vi "Inverse Filter Demo-1.vi"() -> ()   [LabVIEW 2015]
uses:
  Utility VIs/Math VIs/FFT x(t) to dB,Degrees (1D).vi
  Utility VIs/Math VIs/Linear to dB (array).vi
  <vilib>/Analysis/NI_AALBase.lvlib
  Utility VIs/Math VIs/dB to Linear (1D).vi
panel:
  out "size(s)":i32
  out "Noise in 2":dbl[](graph)
  in  "T (s)":dbl
  in  "Fs (Hz)":dbl
  out "Noise out":cluster{"Frequency (Hz)":dbl[], "Mag":dbl[]}(graph)
  out "Noise in":dbl[](graph)
  out "Calibration":T1(graph)
  in  "Calibration file":path
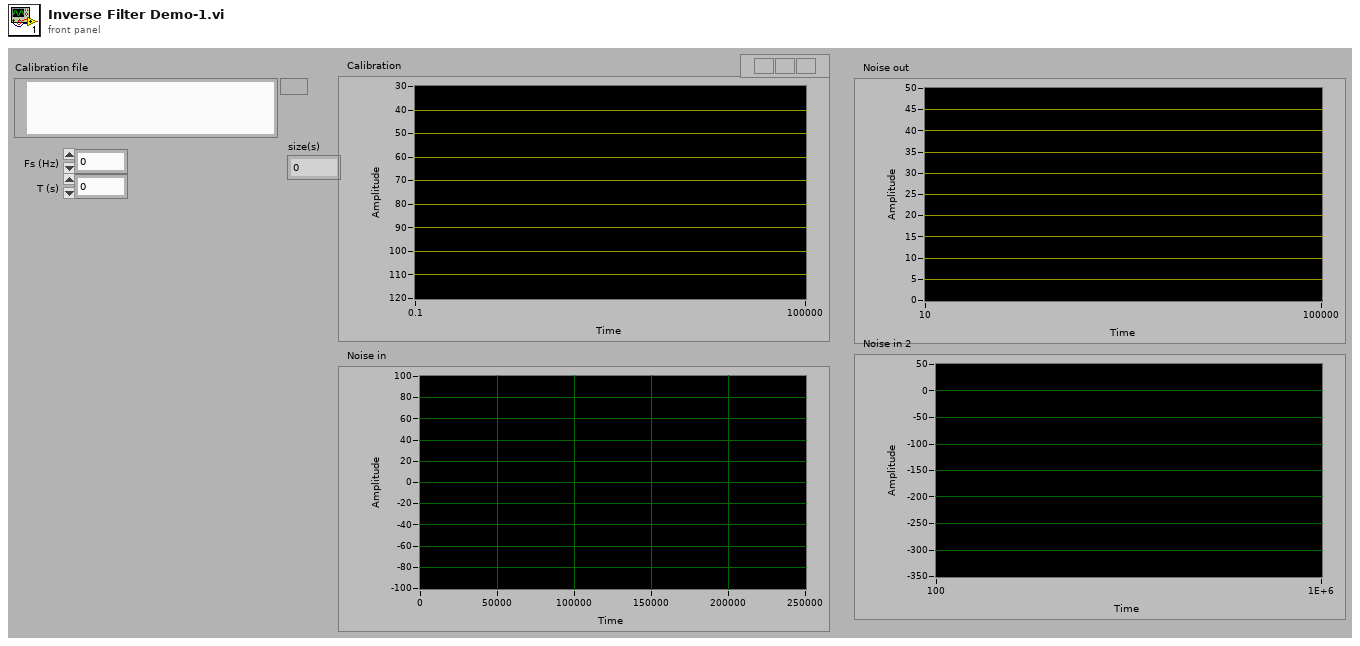
[diagram p1: front panel]
types:
  T1 = cluster{"Interp Freq (Hz)":dbl[], "Interp Magnitude (dB)":dbl[]}[]
  T2 = cluster{"Interp Freq (Hz)":dbl[], "Interp Magnitude (dB)":dbl[]}
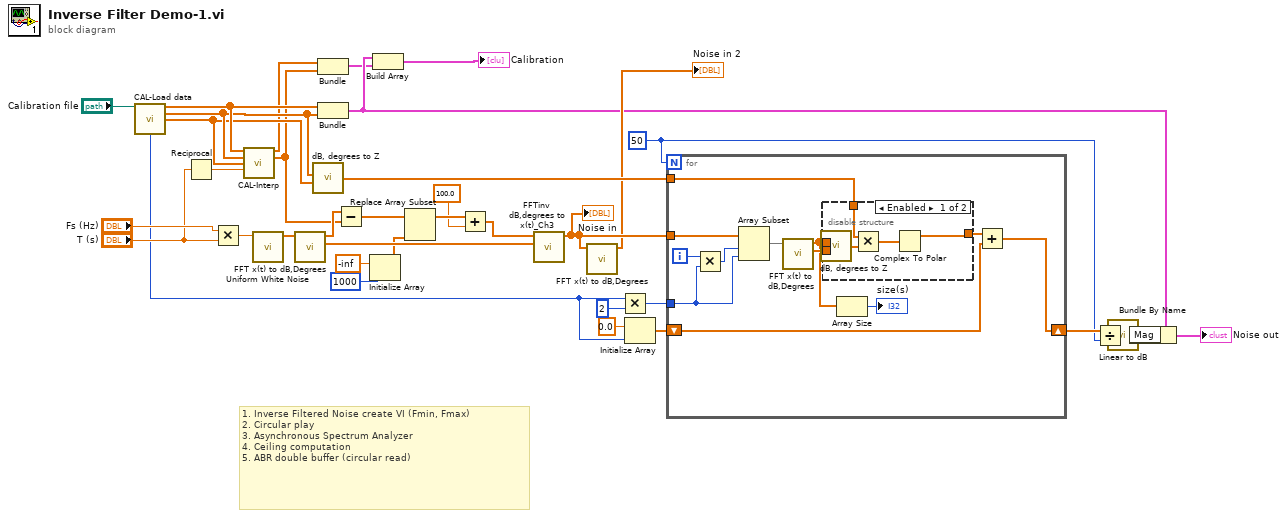
[diagram p0: block diagram]
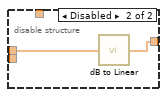
[diagram p2: hidden frame]
diagram:
  w19 = 50
  # "1. Inverse Filtered Noise create VI (Fmin, Fmax)\n2. Circular play\n3. Asynchronous Spectrum Analyzer\n4. Ceiling computation\n5. ABR double buffer (circular read)"
  n1 = call "CAL-Load data.vi"("user path"="Calibration file") -> ("Frequency (Hz)"=w31:dbl[], "Mag"=w28:dbl[], "Phase"=w27:dbl[], "npts"=w21:i32)  [unwired: 7 in, 4 out]
  n2 = Reciprocal(x="T (s)") -> (1/x=w6:dbl)
  n3 = Multiply(x="Fs (Hz)", y="T (s)") -> (x*y=w32:dbl)
  n4 = call "CAL-Interp.vi"("Frequency (Hz)"=w31, "Magnitude (dB)"=w28, "Phase (degrees)"=w27, "df (Hz)"=w6) -> ("Interp Freq (Hz)"=w5:dbl[], "Interp Magnitude (dB)"=w4:dbl[])  [unwired: 8 in, 2 out]
  n5 = call <vilib>:"Uniform White Noise.vi"("samples"=w32) -> ("uniform white noise"=w35:dbl[])  [unwired: 9 in, 1 out]
  n6 = call-poly "FFT x(t) to dB,Degrees.vi"("X"=w35) -> ("+Freq Phase of FFT (degrees)"=w29:dbl[], "+Freq. Mag of FFT (dB rms)"=w34:dbl[])  [unwired: 8 in, 1 out]
  n7 = call "dB, degrees to Z.vi"("Magnitude (dB)"=w28, "Phase (degrees)"=w27) -> ("Z"=w26:cdb[])  [unwired: 5 in]
  n8 = Bundle("Interp Freq (Hz)"=w5, "Interp Magnitude (dB)"=w4) -> (w2:T2)  [unwired: 1 in]
  n9 = Bundle("Frequency (Hz)"=w31, "Mag"=w28) -> (w3:cluster{"Frequency (Hz)":dbl[], "Mag":dbl[]})  [unwired: 1 in]
  n10 = Subtract(x=w34, y=w4) -> (x-y=w16:dbl[])
  n11 = Initialize Array(-inf ("element"), 1000 ("dimension size")) -> (w12:dbl[])
  n12 = Build Array(w3, w2) -> (→"Calibration":T1)
  n13 = Replace Array Subset(array=w16, new element=w12) -> (w15:dbl[])  [unwired: 1 in]
  n14 = Add(x=w15, y=100.0 ("element")) -> (x+y=w11:dbl[])
  n15 = call "FFTinv dB,degrees to x(t)_Ch3.vi"("+Freq Phase of FFT (degrees)"=w29, "+Freq. Mag of FFT (rms dB)"=w11) -> ("X(t)"=w9:dbl[])  [unwired: 8 in, 1 out]
  "Noise in" <- w9
  n16 = call-poly "FFT x(t) to dB,Degrees.vi"("X"=w9) -> ("+Freq. Mag of FFT (dB rms)"=→"Noise in 2":dbl[])  [unwired: 8 in, 2 out]
  n17 = Multiply(x=w21, y=2) -> (x*y=w25:i32)
  n18 = Initialize Array(0.0 ("element"), w21) -> (w23:dbl[])
  n19 = for {
    N: w19 -> [_]
    tunnel: w9 -> [w48]
    tunnel: w25 -> [w46]
    tunnel: w26 -> [w42]
    shift-right: [w40] -> w20
    shift-left: w23 -> [w39]
    i -> [w47]
    n20 = Multiply(x=w47, y=w46) -> (x*y=w45:i32)
    n21 = Array Subset(array=w48, index=w45, length=w46) -> (w44:dbl[])
    n22 = call-poly "FFT x(t) to dB,Degrees.vi"("X"=w44) -> ("+Freq Phase of FFT (degrees)"=w43:dbl[], "+Freq. Mag of FFT (dB rms)"=w38:dbl[])  [unwired: 8 in, 1 out]
    n23 = disable-structure shown="Enabled" {
      disable-tunnel: w38 -> [w54 w56]
      disable-tunnel: w43 -> [w53 _]
      disable-tunnel: w42 -> [w51 _]
      disable-tunnel: [w49 w55] -> w41
      frame Enabled {
        n24 = call "dB, degrees to Z.vi"("Magnitude (dB)"=w54, "Phase (degrees)"=w53) -> ("Z"=w52:cdb[])  [unwired: 5 in]
        n25 = Multiply(x=w51, y=w52) -> (x*y=w50:cdb[])
        n26 = Complex To Polar(r * e^(i*theta)=w50) -> (r=w49:dbl[])  [unwired: 1 out]
      }
      frame Disabled {
        n27 = call-poly "dB to Linear.vi"("dB"=w56) -> ("linear"=w55:dbl[])
      }
    }
    n28 = Array Size(array=w38) -> (size(s)=→"size(s)":i32)
    n29 = Add(x=w41, y=w39) -> (x+y=w40:dbl[])
  }
  n30 = Divide(x=w20, y=w19) -> (x/y=w18:dbl[])
  n31 = call-poly "Linear to dB.vi"("linear"=w18) -> ("dB"=w7:dbl[])
  n32 = Bundle By Name(cluster=w3, "Mag"=w7) -> (→"Noise out":cluster{"Frequency (Hz)":dbl[], "Mag":dbl[]})
